vi "Meas Single Record.vi"(7 "sequence item":T1, 8 "error in":errorcluster, 10 "binary data file path (no ext.)":path, 11 "adc session in":T10={"niScope"={"channel cfg"=[], "sessions"=[], "multi cards"=FALSE, "channels"=0, "type"=enum."n/a", "memory [B/chn]"=0, "ext. clock [Hz]"=0.0, "samples count"=0, "use streaming"=FALSE, "proc setup"={"packet size [smpl]"=0, "current timeout [s]"=0.0, "blk2blk timeout [s]"=0.0, "event time"=timestamp(0 s since 1904-01-01), "temp sampl T [s]"=0.0, "data queue"=refnum, "stop notifier"=refnum, "proc ref"=refnum}, "sample width [B]"=0, "ranges [V]"=[], "trigger setup"={"coupling"=1, "level [V]"=0.0, "slope"=0, "mode"=enum."Immediate"}, "fs [Hz]"=0.0, "bitres [bit]"=0, "clock source"=enum."VAL_NO_SOURCE"}, "3458A"={"channels"=[], "sync unit"={"VISA"="", "type"=enum."Picotest U6200A"}, "awg unit"={"type"=enum."Agilent 331xxA to 332xxA", "VISA"="", "enable 10MHz ref"=FALSE}, "sync mode"=enum."MASTER-SLAVE, MASTER clocked by TIMER", "streaming mode"=FALSE, "idn mode"=enum."Auto", "sampling mode"=enum."DCV", "Ts [s]"=0.0, "sample memory [B]"=0, "proc setup"={"channel id"=0, "packet size [smpl]"=0, "current timeout [s]"=0.0, "blk2blk timeout [s]"=0.0, "event time"=timestamp(0 s since 1904-01-01), "stop notifier"=refnum, "data queues"=[], "proc refs"=[], "bus semaphore"=refnum}, "sample size [B]"=0, "sample count"=0, "aux data"={"channel id"=0, "valid?"=[], "gain [V]"=[], "timestamp [s]"=[], "Ts [s]"=0.0, "abs timestamp"=timestamp(0 s since 1904-01-01), "t [deg C]"=[], "multiplex timestamp [s]"=-1.0, "only multiplex?"=FALSE, "multiplex smpl offset"=0}, "ranges [V]"=[], "aperture [s]"=0.0, "LEVEL trigger"={"edge"=enum."POS", "level [V]"=0.0, "coupling"=enum."DC"}, "trigger mode"=enum."AUTO", "measure temp.?"=FALSE, "disp mesages"=[], "shared bus?"=FALSE, "disable display?"=FALSE, "aper mode"=enum."Manual", "aper rules"=[], "multiplex"={"cycles"=0, "delay [s]"=0.0, "enabled"=FALSE, "overhead [s]"=1.0, "tot smpls"=0}}, "dsdll"={"dsdll"={"dsdll path"=path "", "dsdll handle"=[], "output devices"=[], "capture devices"=[]}, "channels"=0, "device id"=0, "channel idns"=[], "proc setup"={"packet size [smpl]"=0, "current timeout [s]"=0.0, "blk2blk timeout [s]"=0.0, "event time"=timestamp(0 s since 1904-01-01), "data queue"=refnum, "stop notifier"=refnum, "proc ref"=refnum}, "samples count"=0, "fs [Hz]"=0.0}, "type"=enum."niScope", "channel idn str"=[], "aux instr idn str"=[], "modified?"=FALSE, "simadc"={"channels"=[], "range [V]"=0.0, "Ts step [s]"=0.0, "time [s]"=0.0, "fs [Hz]"=0.0, "count"=0, "smpl offset"=0, "set count"=0, "bit res"=0}, "force rst?"=FALSE, "exit mode"=enum."Immediate reset", "exit dly"=0.0, "exit tmr"=timestamp(0 s since 1904-01-01), "busy?"=FALSE, "accessed?"=FALSE, "multiplex"={"Type"=enum."Dummy", "gen com ssn"={"visa"="", "primary"=enum."None", "secondary"=enum."None", "channels"=[]}, "delay before [s]"=0.0, "delay post [s]"=0.0, "sequence"=[], "enabled"=FALSE, "ref timestamp [s]"=0.0, "idn string"="", "dev niScope"="", "niScope idx"=0}} {"3458A"."channels"."Range [Vpk]" min=0.0; "niScope"."trigger setup"."level [V]" format="%.2f"; "niScope"."trigger setup"."coupling" items=["AC"=0, "DC"=1, "HF Reject"=3, "LF Reject"=4, "AC Plus HF Reject"=1001]; "niScope"."channel cfg"."Range [Vpk]" min=0.0; "niScope"."channel cfg"."Channel" min=0}) -> (0 "error out":errorcluster, 1 "aborted?":bool, 2 "aux data":T9, 3 "adc session out":T10={"niScope"={"channel cfg"=[], "sessions"=[], "multi cards"=FALSE, "channels"=0, "type"=enum."n/a", "memory [B/chn]"=0, "ext. clock [Hz]"=0.0, "samples count"=0, "use streaming"=FALSE, "proc setup"={"packet size [smpl]"=0, "current timeout [s]"=0.0, "blk2blk timeout [s]"=0.0, "event time"=timestamp(0 s since 1904-01-01), "temp sampl T [s]"=0.0, "data queue"=refnum, "stop notifier"=refnum, "proc ref"=refnum}, "sample width [B]"=0, "ranges [V]"=[], "trigger setup"={"coupling"=1, "level [V]"=0.0, "slope"=0, "mode"=enum."Immediate"}, "fs [Hz]"=0.0, "bitres [bit]"=0, "clock source"=enum."VAL_NO_SOURCE"}, "3458A"={"channels"=[], "sync unit"={"VISA"="", "type"=enum."Picotest U6200A"}, "awg unit"={"type"=enum."Agilent 331xxA to 332xxA", "VISA"="", "enable 10MHz ref"=FALSE}, "sync mode"=enum."MASTER-SLAVE, MASTER clocked by TIMER", "streaming mode"=FALSE, "idn mode"=enum."Auto", "sampling mode"=enum."DCV", "Ts [s]"=0.0, "sample memory [B]"=0, "proc setup"={"channel id"=0, "packet size [smpl]"=0, "current timeout [s]"=0.0, "blk2blk timeout [s]"=0.0, "event time"=timestamp(0 s since 1904-01-01), "stop notifier"=refnum, "data queues"=[], "proc refs"=[], "bus semaphore"=refnum}, "sample size [B]"=0, "sample count"=0, "aux data"={"channel id"=0, "valid?"=[], "gain [V]"=[], "timestamp [s]"=[], "Ts [s]"=0.0, "abs timestamp"=timestamp(0 s since 1904-01-01), "t [deg C]"=[], "multiplex timestamp [s]"=-1.0, "only multiplex?"=FALSE, "multiplex smpl offset"=0}, "ranges [V]"=[], "aperture [s]"=0.0, "LEVEL trigger"={"edge"=enum."POS", "level [V]"=0.0, "coupling"=enum."DC"}, "trigger mode"=enum."AUTO", "measure temp.?"=FALSE, "disp mesages"=[], "shared bus?"=FALSE, "disable display?"=FALSE, "aper mode"=enum."Manual", "aper rules"=[], "multiplex"={"cycles"=0, "delay [s]"=0.0, "enabled"=FALSE, "overhead [s]"=1.0, "tot smpls"=0}}, "dsdll"={"dsdll"={"dsdll path"=path "", "dsdll handle"=[], "output devices"=[], "capture devices"=[]}, "channels"=0, "device id"=0, "channel idns"=[], "proc setup"={"packet size [smpl]"=0, "current timeout [s]"=0.0, "blk2blk timeout [s]"=0.0, "event time"=timestamp(0 s since 1904-01-01), "data queue"=refnum, "stop notifier"=refnum, "proc ref"=refnum}, "samples count"=0, "fs [Hz]"=0.0}, "type"=enum."niScope", "channel idn str"=[], "aux instr idn str"=[], "modified?"=FALSE, "simadc"={"channels"=[], "range [V]"=0.0, "Ts step [s]"=0.0, "time [s]"=0.0, "fs [Hz]"=0.0, "count"=0, "smpl offset"=0, "set count"=0, "bit res"=0}, "force rst?"=FALSE, "exit mode"=enum."Immediate reset", "exit dly"=0.0, "exit tmr"=timestamp(0 s since 1904-01-01), "busy?"=FALSE, "accessed?"=FALSE, "multiplex"={"Type"=enum."Dummy", "gen com ssn"={"visa"="", "primary"=enum."None", "secondary"=enum."None", "channels"=[]}, "delay before [s]"=0.0, "delay post [s]"=0.0, "sequence"=[], "enabled"=FALSE, "ref timestamp [s]"=0.0, "idn string"="", "dev niScope"="", "niScope idx"=0}} {"3458A"."channels"."Range [Vpk]" min=0.0; "niScope"."trigger setup"."level [V]" format="%.2f"; "niScope"."trigger setup"."coupling" items=["AC"=0, "DC"=1, "HF Reject"=3, "LF Reject"=4, "AC Plus HF Reject"=1001]; "niScope"."channel cfg"."Range [Vpk]" min=0.0; "niScope"."channel cfg"."Channel" min=0}, 4 "acquired samples per channel":i64, 6 "record segments info":T8[](array[typedef]))   [LabVIEW 2013]
doc: "This VI initiates sampling of one record with current setup of ADC. It streams the sample data to MAT file of a given path (without extension). The VI also appends logged temperatures to the MAT file. It will return ADC auxiliary data which are valid only if flag 'valid?' in the cluster is True (that should happen all the time except when the sampling was aborted for whatever reason). The VI responds to global stop button called 'btn stop' - it will abort sampling when it is in True state.\n\nIn time multiplexing mode the samples from particular cycles are stored as one stream to the MAT file. Along with them the VI returns 'multiplexing sample offsets', which are zero-based offsets of first sample for each multiplexing cycle."
uses:
  adc/ADC Session.ctl
  drivers/niScope/niScope Session.ctl
  drivers/niScope/niScope Virtual Channel Config.ctl
  drivers/niScope/niScope Virtual Channel Mode.ctl
  drivers/niScope/niScope Virtual Channel Input Z.ctl
  drivers/niScope/niScope Virtual Channel Coupling.ctl
  drivers/niScope/niScope Type.ctl
  drivers/niScope/niScope Digitizing Process Options.ctl
  drivers/niScope/niScope Data Packet.ctl
  drivers/niScope/niScope Trigger Setup.ctl
  <instrlib>/niScope/Controls/niScope trigger coupling.ctl
  <instrlib>/niScope/Controls/niScope trigger slope.ctl
  drivers/niScope/niScope Reference Clock.ctl
  drivers/DMM/3458A Digitizer Session.ctl
  drivers/DMM/3458A Virtual Channel Config.ctl
  drivers/Counter/Counter Session.ctl
  drivers/Counter/Counter Type.ctl
  drivers/AWG/AWG Session.ctl
  drivers/AWG/AWG Type.ctl
  drivers/DMM/3458A Sync Mode.ctl
  drivers/DMM/3458A Idn Mode.ctl
  drivers/DMM/3458A Digitizing Low Levels/Configure/Sampling Mode.ctl
  drivers/DMM/3458A Digitizing Process Options.ctl
  drivers/DMM/3458A Data Packet.ctl
  drivers/DMM/3458A Aux Record Data.ctl
  drivers/DMM/3458A Digitizing Low Levels/Configure/Level Setup.ctl
  drivers/DMM/3458A Digitizing Low Levels/Configure/First Sample Trigger.ctl
  drivers/DMM/3458A Aperture Selection Mode.ctl
  drivers/DMM/3458A Multiplexing Config.ctl
  drivers/dsdll/DSDLL Session.ctl
  drivers/dsdll/dsdll.lvlibp/dsdll_instance.ctl
  drivers/dsdll/dsdll.lvlibp/dsdll_device_record.ctl
  drivers/dsdll/DSDLL Process Config.ctl
  drivers/dsdll/DSDLL Data Packet.ctl
  adc/ADC Type.ctl
  drivers/simulated_adc/SimAdc Config.ctl
  drivers/simulated_adc/SimAdc Channel Cfg.ctl
  adc/ADC On Close Action.ctl
  adc/Multiplexer/MPX Session.ctl
  adc/Multiplexer/MPX Type.ctl
  drivers/Multiplexers/Generic COM/GCOMM Session.ctl
  drivers/Multiplexers/Generic COM/GCOMM Signal.ctl
  drivers/Multiplexers/Generic COM/GCOMM Virtual Channel.ctl
  drivers/Multiplexers/Generic COM/GCOMM Logic State.ctl
  adc/ADC Aux Data.ctl
  adc/Multiplexer/MPX Record Segment Info.ctl
  Meas Sequence Item.ctl
  Meas Sampling Configuration.ctl
  adc/ADC Trig Config.ctl
  adc/ADC Trig Mode Source.ctl
  adc/ADC Trig Coupling.ctl
  adc/ADC Trig Slope.ctl
  processing/QWTB/Meas Proc QWTB Algorithm Parameter Data.ctl
  octave/mat/MAT Type Representation.ctl
  varilib/SGUI Assign Multiple Strings With Tags By Label.vi
  varilib/varilib.lvlib
  drivers/niScope/niScope Virtual Digitizer.lvlib
  drivers/DMM/3458A Virtual Digitizer.lvlib
  drivers/Counter/Counter.lvlib
  drivers/AWG/AWG.lvlib
  drivers/DMM/3458A Digitizing Low Levels/3458A Digitizing Low Levels.lvlib
  drivers/dsdll/dsdll.lvlibp
  drivers/dsdll/DSDLL Virtual Digitizer.lvlib
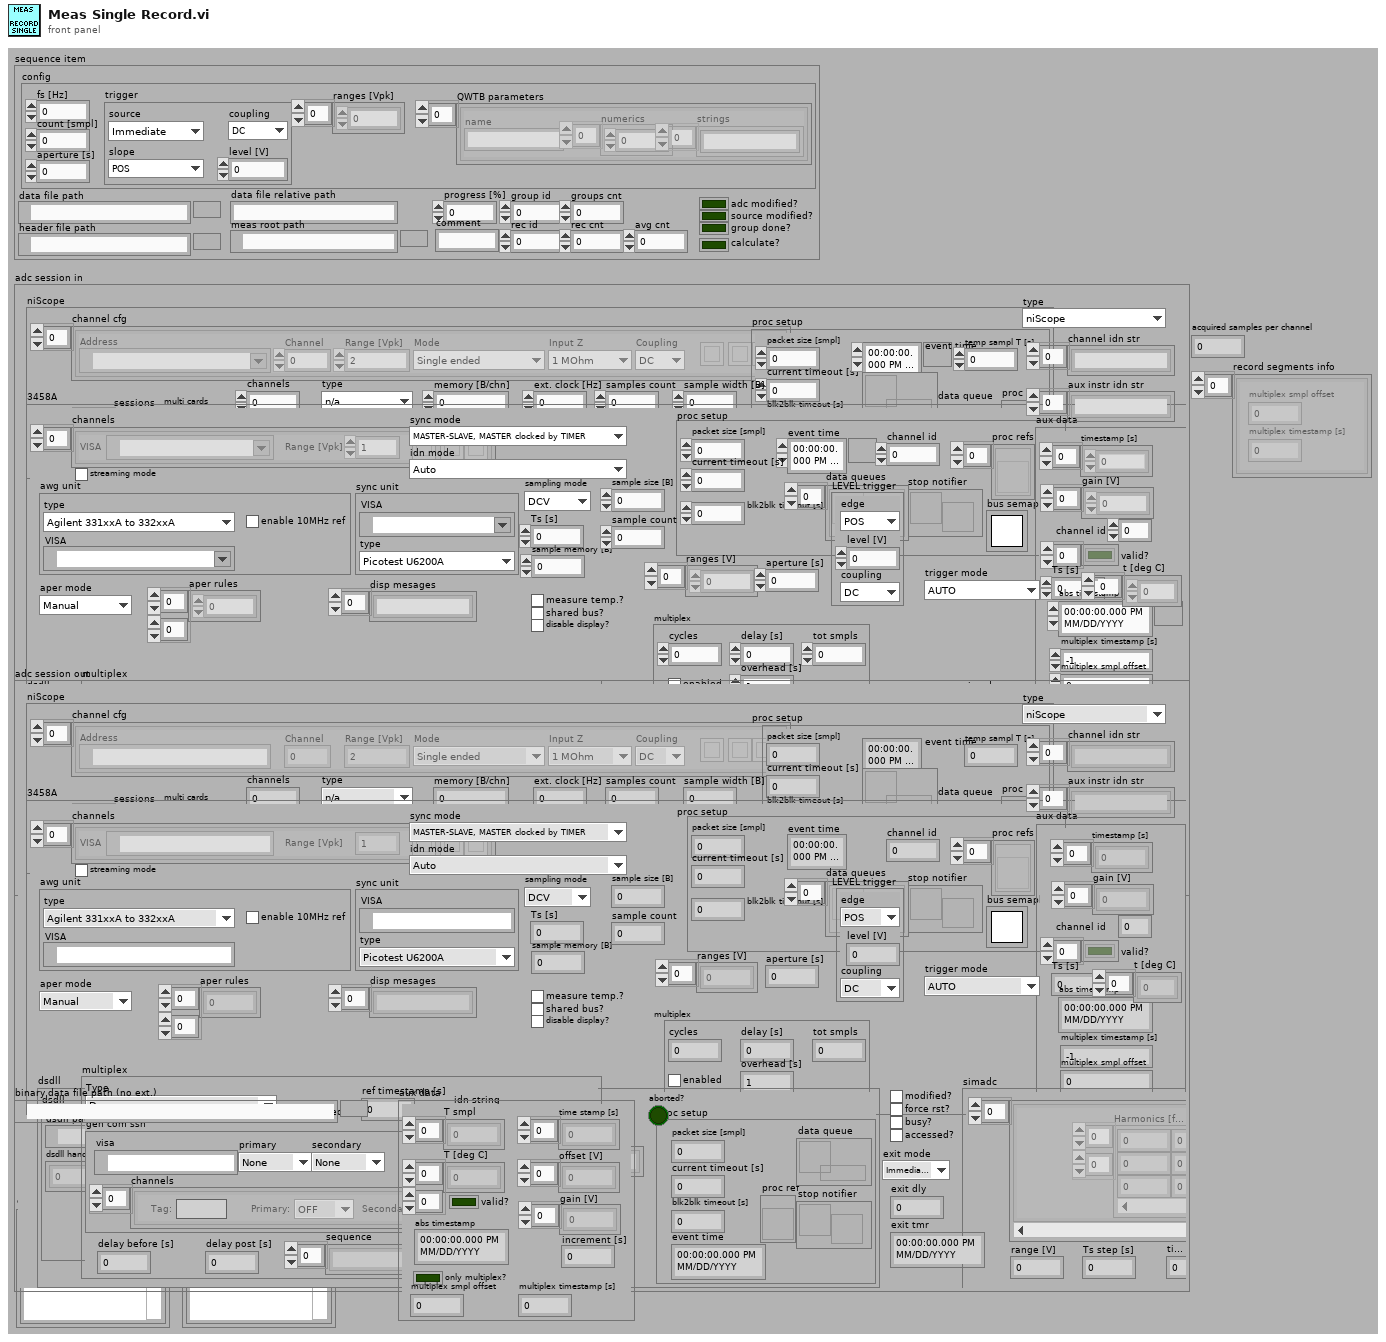
[diagram p1: front panel]
types:
  T1 = typedef "Meas Sequence Item.ctl" = cluster{"config":T2, "data file path":path, "header file path":path, "group id":i32, "rec id":i32, "group done?":bool, "adc modified?":bool, "source modified?":bool, "progress [%]":dbl, "groups cnt":i32, "rec cnt":i32, "data file relative path":string, "meas root path":path, "calculate?":bool, "comment":string, "avg cnt":i32}
  T2 = typedef "Meas Sampling Configuration.ctl" = cluster{"fs [Hz]":dbl, "count [smpl]":i64, "aperture [s]":dbl, "trigger":T3, "ranges [Vpk]":dbl[], "QWTB parameters":T7[]}
  T3 = typedef "ADC Trig Config.ctl" = cluster{"source":T4, "level [V]":dbl, "coupling":T5, "slope":T6}
  T4 = typedef "ADC Trig Mode Source.ctl" = enum16{"Immediate", "External", "Level"}
  T5 = typedef "ADC Trig Coupling.ctl" = enum16{"DC", "AC"}
  T6 = typedef "ADC Trig Slope.ctl" = enum16{"POS", "NEG"}
  T7 = typedef "Meas Proc QWTB Algorithm Parameter Data.ctl" = cluster{"name":string, "numerics":dbl[], "strings":string[]}
  T8 = typedef "MPX Record Segment Info.ctl" = cluster{"multiplex smpl offset":i64, "multiplex timestamp [s]":dbl}
  T9 = typedef "ADC Aux Data.ctl" = cluster{"offset [V]":dbl[], "gain [V]":dbl[], "time stamp [s]":dbl[], "increment [s]":dbl, "T smpl":i64[], "T [deg C]":dbl[][], "valid?":bool, "abs timestamp":timestamp, "only multiplex?":bool, "multiplex smpl offset":i64, "multiplex timestamp [s]":dbl}
  T10 = typedef "ADC Session.ctl" = cluster{"niScope":T11, "3458A":T22, "dsdll":T38, "type":T42, "channel idn str":string[], "aux instr idn str":string[], "modified?":bool, "simadc":T43, "force rst?":bool, "exit mode":T45, "exit dly":dbl, "exit tmr":timestamp, "busy?":bool, "accessed?":bool, "multiplex":T46}
  T11 = typedef "niScope Virtual Digitizer.lvlib/niScope Session.ctl" = cluster{"channel cfg":T12[], "sessions":refnum<k20>[], "multi cards":bool, "channels":i32, "type":T16, "memory [B/chn]":i32, "ext. clock [Hz]":dbl, "samples count":i64, "use streaming":bool, "proc setup":T17, "sample width [B]":i32, "ranges [V]":dbl[], "trigger setup":T18, "fs [Hz]":dbl, "bitres [bit]":i32, "clock source":T21}
  T12 = typedef "niScope Virtual Digitizer.lvlib/niScope Virtual Channel Config.ctl" = cluster{"Address":refnum<k15>, "Channel":i32, "Mode":T13, "Input Z":T14, "Coupling":T15, "Range [Vpk]":dbl, "btn clr":bool, "btn up":bool, "btn down":bool}
  T13 = typedef "niScope Virtual Digitizer.lvlib/niScope Virtual Channel Mode.ctl" = enum16{"Single ended", "Unbal. differential", "Differential"}
  T14 = typedef "niScope Virtual Digitizer.lvlib/niScope Virtual Channel Input Z.ctl" = enum16{"1 MOhm", "50 Ohm"}
  T15 = typedef "niScope Virtual Digitizer.lvlib/niScope Virtual Channel Coupling.ctl" = enum16{"AC", "DC", "GND"}
  T16 = typedef "niScope Virtual Digitizer.lvlib/niScope Type.ctl" = enum16{"n/a", "5922"}
  T17 = typedef "niScope Virtual Digitizer.lvlib/niScope Digitizing Process Options.ctl" = cluster{"packet size [smpl]":i64, "current timeout [s]":dbl, "blk2blk timeout [s]":dbl, "event time":timestamp, "temp sampl T [s]":dbl, "data queue":refnum<queue>, "stop notifier":refnum<notifier>, "proc ref":refnum<vi>}
  T18 = typedef "niScope Virtual Digitizer.lvlib/niScope Trigger Setup.ctl" = cluster{"coupling":T19, "level [V]":dbl, "slope":T20, "mode":enum16{"Immediate", "External", "Level"}}
  T19 = typedef "niScope trigger coupling.ctl" = u16
  T20 = typedef "niScope trigger slope.ctl" = i32
  T21 = typedef "niScope Virtual Digitizer.lvlib/niScope Reference Clock.ctl" = enum16{"VAL_NO_SOURCE", "VAL_CLK_IN", "VAL_PXI_CLOCK", "VAL_EXTERNAL"}
  T22 = typedef "3458A Virtual Digitizer.lvlib/3458A Digitizer Session.ctl" = cluster{"channels":T23[], "sync unit":T24, "awg unit":T26, "sync mode":T28, "streaming mode":bool, "idn mode":T29, "sampling mode":T30, "Ts [s]":dbl, "sample memory [B]":i32, "proc setup":T31, "sample size [B]":i32, "sample count":i32, "aux data":T33, "ranges [V]":dbl[], "aperture [s]":dbl, "LEVEL trigger":T34, "trigger mode":T35, "measure temp.?":bool, "disp mesages":string[], "shared bus?":bool, "disable display?":bool, "aper mode":T36, "aper rules":dbl[][], "multiplex":T37}
  T23 = typedef "3458A Virtual Digitizer.lvlib/3458A Virtual Channel Config.ctl" = cluster{"VISA":refnum<visa-resource-name>, "Range [Vpk]":dbl, "btn clr":bool, "btn up":bool, "btn down":bool}
  T24 = typedef "Counter.lvlib/Counter Session.ctl" = cluster{"VISA":refnum<visa-resource-name>, "type":T25}
  T25 = typedef "Counter.lvlib/Counter Type.ctl" = enum16{"Picotest U6200A", "dummy"}
  T26 = typedef "AWG.lvlib/AWG Session.ctl" = cluster{"type":T27, "VISA":refnum<visa-resource-name>, "enable 10MHz ref":bool}
  T27 = typedef "AWG.lvlib/AWG Type.ctl" = enum16{"Agilent 331xxA to 332xxA", "Agilent 335xxA to 336xxA", "Tektronix AFG3101C", "dummy"}
  T28 = typedef "3458A Virtual Digitizer.lvlib/3458A Sync Mode.ctl" = enum16{"MASTER-SLAVE, MASTER clocked by TIMER", "MASTER-SLAVE, MASTER clocked by AWG", "ALL clocked by AWG", "MASTER-SLAVE, ALL clocked by TIMER", "ALL clocked by AWG with DFLL"}
  T29 = typedef "3458A Virtual Digitizer.lvlib/3458A Idn Mode.ctl" = enum16{"Auto", "Sequential (chn A, chn B, ...)", "From calibration string"}
  T30 = typedef "3458A Virtual Digitizer.lvlib/3458A Digitizing Low Levels.lvlib/Sampling Mode.ctl" = enum16{"DCV", "DSDC", "DSAC"}
  T31 = typedef "3458A Virtual Digitizer.lvlib/3458A Digitizing Process Options.ctl" = cluster{"channel id":i32, "packet size [smpl]":i32, "current timeout [s]":dbl, "blk2blk timeout [s]":dbl, "event time":timestamp, "stop notifier":refnum<notifier>, "data queues":refnum<queue>[], "proc refs":refnum<vi>[], "bus semaphore":T32}
  T32 = typedef "Semaphore RefNum" = refnum<k1>
  T33 = typedef "3458A Virtual Digitizer.lvlib/3458A Aux Record Data.ctl" = cluster{"channel id":i32, "valid?":bool[], "gain [V]":dbl[], "timestamp [s]":dbl[], "Ts [s]":dbl, "abs timestamp":timestamp, "t [deg C]":dbl[], "multiplex timestamp [s]":dbl, "only multiplex?":bool, "multiplex smpl offset":i64}
  T34 = typedef "3458A Virtual Digitizer.lvlib/3458A Digitizing Low Levels.lvlib/Level Setup.ctl" = cluster{"edge":enum16{"POS", "NEG"}, "level [V]":dbl, "coupling":enum16{"DC", "AC"}}
  T35 = typedef "3458A Virtual Digitizer.lvlib/3458A Digitizing Low Levels.lvlib/First Sample Trigger.ctl" = enum16{"AUTO", "EXT", "SYN", "SGL", "HOLD", "LEVEL"}
  T36 = typedef "3458A Virtual Digitizer.lvlib/3458A Aperture Selection Mode.ctl" = enum16{"Manual", "Maximum", "Table"}
  T37 = typedef "3458A Multiplexing Config.ctl" = cluster{"cycles":i32, "delay [s]":dbl, "enabled":bool, "overhead [s]":dbl, "tot smpls":i64}
  T38 = typedef "DSDLL Virtual Digitizer.lvlib/DSDLL Session.ctl" = cluster{"dsdll":T39, "channels":i32, "device id":i32, "channel idns":string[], "proc setup":T41, "samples count":i32, "fs [Hz]":dbl}
  T39 = typedef "dsdll.lvlibp/dsdll_instance.ctl" = cluster{"dsdll path":path, "dsdll handle":u8[], "output devices":T40[], "capture devices":T40[]}
  T40 = typedef "dsdll.lvlibp/dsdll_device_record.ctl" = cluster{"guid":u8[], "name":string}
  T41 = typedef "DSDLL Virtual Digitizer.lvlib/DSDLL Process Config.ctl" = cluster{"packet size [smpl]":i32, "current timeout [s]":dbl, "blk2blk timeout [s]":dbl, "event time":timestamp, "data queue":refnum<queue>, "stop notifier":refnum<notifier>, "proc ref":refnum<vi>}
  T42 = typedef "ADC Type.ctl" = enum16{"niScope", "3458A", "DirectSound DLL", "dummy"}
  T43 = typedef "SimAdc Config.ctl" = cluster{"channels":T44[], "range [V]":dbl, "Ts step [s]":dbl, "time [s]":dbl, "fs [Hz]":dbl, "count":i64, "smpl offset":i64, "set count":i64, "bit res":i32}
  T44 = typedef "SimAdc Channel Cfg.ctl" = cluster{"harmonics":dbl[][], "btn clear":bool, "noise":dbl, "fundamental [Hz]":dbl}
  T45 = typedef "ADC On Close Action.ctl" = enum16{"Immediate reset", "Delayed reset"}
  T46 = typedef "MPX Session.ctl" = cluster{"Type":T47, "gen com ssn":T48, "delay before [s]":dbl, "delay post [s]":dbl, "sequence":string[], "enabled":bool, "ref timestamp [s]":dbl, "idn string":string, "dev niScope":refnum<k15>, "niScope idx":i32}
  T47 = typedef "MPX Type.ctl" = enum16{"Dummy", "Generic - COM port", "Generic - niScope PFI"}
  T48 = typedef "GCOMM Session.ctl" = cluster{"visa":refnum<visa-resource-name>, "primary":T49, "secondary":T49, "channels":T50[]}
  T49 = typedef "GCOMM Signal.ctl" = enum16{"None", "DTR", "RTS"}
  T50 = typedef "GCOMM Virtual Channel.ctl" = cluster{"Primary:":T51, "Secondary:":T51, "btn clr":bool, "btn up":bool, "btn down":bool, "Tag:":string}
  T51 = typedef "GCOMM Logic State.ctl" = enum16{"OFF", "ON"}
  T52 = typedef "MAT Type Representation.ctl" = enum16{"DBL", "SGL", "I32", "I16", "U16", "U8", "CDB", "CSG", "STR"}
  T53 = typedef "ADC Current Configuration.ctl" = cluster{"count [smpl]":i64, "channels count":i32, "fs [Hz]":dbl, "ranges [V]":dbl[], "trigger":T3, "ext freq. locked?":bool, "streaming on?":bool, "is int16?":bool, "bitres":i32}
  T54 = typedef "Meas Samples Stream.ctl" = cluster{"file ref":refnum<file>, "data offset [B]":i64, "var offset [B]":i64, "data type":T52, "written smpls":i64, "channels":i64}
  T55 = typedef "ADC Data Packet.ctl" = cluster{"int32":i32[][], "int16":i16[][], "offset [smpl]":i64, "count [smpl]":i32, "is int16?":bool, "all done?":bool, "sampling?":bool, "instr buffer [%]":dbl, "queue buffer [%]":dbl, "valid?":bool}
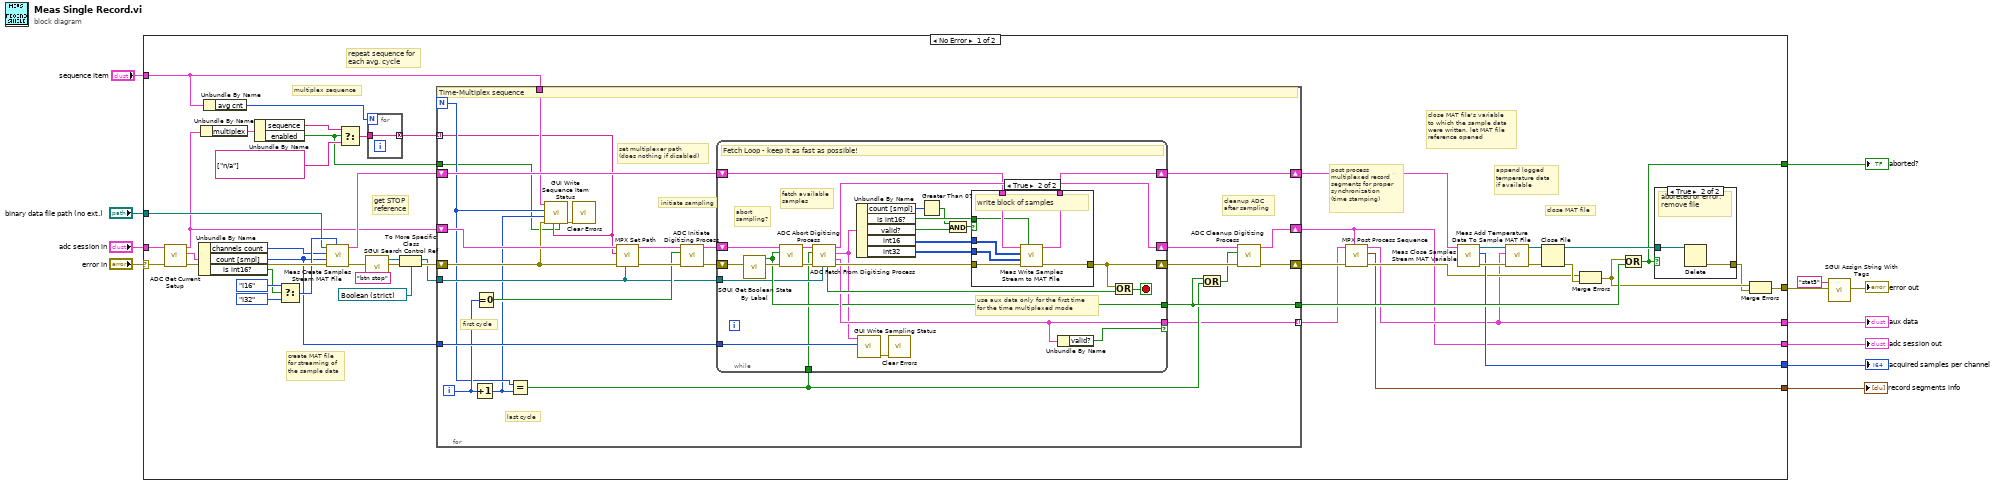
[diagram p0: block diagram]
diagram:
  n1 = case shown="No Error" "error in" {
    selector: "error in" -> [w46 w126]
    tunnel: "adc session in" -> [w59 w125]
    tunnel: "binary data file path (no ext.)" -> [w54 _]
    tunnel: [w41 w126] -> w5
    tunnel: [w18 w125] -> w9
    tunnel: [w20 _] -> w8
    tunnel: [w40 _] -> w7
    tunnel: [w37 _] -> w6
    tunnel: [w19 _] -> w2
    tunnel: "sequence item" -> [w14 _]
    frame No Error {
      # "repeat sequence for\neach avg. cycle"
      # "post process\nmultiplexed record\nsegments for proper\nsynchronization\n(time stamping)"
      # "get STOP\nreference"
      # "multiplex sequence"
      # "close MAT file"
      # "append logged\ntemperature data\nif available"
      # "close MAT file's variable\nto which the sample data\nwere written, let MAT file\nreference opened"
      # "create MAT file\nfor streaming of\nthe sample data"
      n2 = call "ADC Get Current Setup.vi"("error in"=w46, "adc session in"=w59) -> ("error out"=w58:errorcluster, "common attributes"=w39:T53, "adc session out"=w34:T10)  [unwired: 6 in, 1 out]
      n3 = Unbundle By Name(w39) -> ("channels count"=w36:i32, "count [smpl]"=w35:i64, "is int16?"=w38:bool)
      n4 = Unbundle By Name(w34) -> ("multiplex"=w33:T46)
      n5 = Unbundle By Name(w14) -> ("avg cnt"=w17:i32)
      n6 = Unbundle By Name(w33) -> ("sequence"=w32:string[], "enabled"=w13:bool)
      n7 = Select(t=MAT_Type_Representation."I16" ("data type"), s=w38, f=MAT_Type_Representation."I32" ("data type")) -> (s? t:f=w55:T52)
      n8 = call "Meas Create Samples Stream MAT File.vi"("data type"=w55, "error in"=w58, "samples count"=w35, "channels count"=w36, "binary data file path"=w54) -> ("error out"=w29:errorcluster, "stream session"=w53:T54)  [unwired: 5 in]
      n9 = Select(t=w32, s=w13, f=string[] ["n/a"]) -> (s? t:f=w16:string[])
      n10 = call "SGUI Search Control Ref.vi"("error in"=w29, "control label (empty)"="btn stop") -> ("error out"=w28:errorcluster, "control ref out"=w26:refnum<vi>)  [unwired: 7 in, 1 out]
      n11 = for {
        N: w17 -> [_]
        tunnel: [w60] -> w15 mode=concatenating
        tunnel: w16 -> [w60]
      }
      n12 = To More Specific Class(target class=refnum<vi> refnum ("OK Button"), reference=w26, error in=w28) -> (specific class reference=w25:refnum<vi>, error out=w27:errorcluster)
      n13 = for {
        N -> [w64]
        tunnel: [w70] -> w21 mode=indexing
        tunnel: [w74] -> w45
        tunnel: w35 -> [w82]
        shift-right: [w83] -> w23
        shift-left: w27 -> [w66]
        shift-right: [w84] -> w18
        shift-left: w34 -> [w69]
        shift-right: [w85] -> w52
        shift-left: w53 -> [w86]
        tunnel: w15 -> [w62] mode=indexing
        tunnel: w25 -> [w75]
        tunnel: w14 -> [w65]
        tunnel: w13 -> [w61]
        i -> [w76]
        # "last cycle"
        # "first cycle"
        # "set multiplexer path\n(does nothing if disabled)"
        # "cleanup ADC \nafter sampling"
        # "initiate sampling"
        # "Time-Multiplex sequence"
        n14 = Increment(x=w76) -> (x+1=w63:i32)
        n15 = Equal To 0?(x=w76) -> (x = 0?=w77:bool)
        n16 = Equal?(x=w64, y=w63) -> (x = y?=w71:bool)
        n17 = call "GUI Write Sequence Item Status.vi"("multiplex enabled (False)"=w61, "multiplex tag"=w62, "error in"=w66, "sub-rec id"=w63, "sub-rec count"=w64, "sequence item"=w65) -> ("error out"=w67:errorcluster)  [unwired: 4 in, 1 out]
        n18 = call <vilib>:"Clear Errors.vi"("error in (no error)"=w67) -> ()  [unwired: 6 in, 1 out]
        n19 = call "MPX Set Path.vi"("stop ref"=w75, "error in"=w66, "path"=w62, "session in"=w69) -> ("error out"=w78:errorcluster, "session out"=w68:T10)  [unwired: 6 in]
        n20 = call "ADC Initiate Digitizing Process.vi"("error in"=w78, "Is first multiplex cycle? (True)"=w77, "adc session in"=w68) -> ("error out"=w72:errorcluster, "adc session out"=w81:T10)  [unwired: 7 in]
        n21 = while {
          shift-right: [w99] -> w80
          shift-left: w72 -> [w113]
          shift-right: [w108] -> w79
          shift-left: w81 -> [w111]
          shift-right: [w103] -> w85
          shift-left: w86 -> [w104]
          tunnel: [w98] -> w70 if=w87
          tunnel: [w97] -> w74
          tunnel: w82 -> [w91]
          tunnel: w75 -> [w89]
          tunnel: w71 -> [w88]
          stop <- w106 stop-if-true
          # "use aux data only for the first time\nfor the time multiplexed mode"
          # "fetch available\nsamples"
          # "abort\nsampling?"
          # "Fetch Loop - keep it as fast as possible!"
          n22 = call "SGUI Get Boolean State By Label.vi"("error in"=w113) -> ("error out"=w112:errorcluster, "binary state out"=w97:bool)  [unwired: 8 in, 1 out]
          n23 = call "ADC Abort Digitizing Process.vi"("error in"=w112, "send abort signal? (True)"=w97, "adc session in"=w111) -> ("error out"=w110:errorcluster, "adc session out"=w109:T10)  [unwired: 7 in]
          n24 = call "ADC Fetch From Digitizing Process.vi"("stop ref"=w89, "error in"=w110, "Is last multiplexing cycle? (True)"=w88, "adc session in"=w109) -> ("error out"=w105:errorcluster, "aux data"=w98:T9, "data packet"=w92:T55, "adc session out"=w108:T10, "fetching done?"=w107:bool)  [unwired: 3 in]
          n25 = Unbundle By Name(w92) -> ("count [smpl]"=w96:i32, "is int16?"=w100:bool, "valid?"=w93:bool, "int16"=w102:i16[][], "int32"=w101:i32[][])
          n26 = call "GUI Write Sampling Status.vi"("total samples"=w91, "data"=w92) -> ("error out"=w90:errorcluster)  [unwired: 9 in]
          n27 = call <vilib>:"Clear Errors.vi"("error in (no error)"=w90) -> ()  [unwired: 6 in, 1 out]
          n28 = Greater Than 0?(x=w96) -> (x > 0?=w94:bool)
          n29 = Compound Arithmetic op=AND(w94, w93) -> (w95:bool)
          n30 = case shown="True" w95 {
            tunnel: w105 -> [w115 w122]
            tunnel: w104 -> [w114 w121]
            tunnel: [w114 w120] -> w103
            tunnel: w102 -> [_ w119]
            tunnel: w101 -> [_ w118]
            tunnel: w100 -> [_ w117]
            tunnel: [w115 w116] -> w99
            frame False {
              # "no data available"
            }
            frame True {
              # "write block of samples"
              n31 = call "Meas Write Samples Stream to MAT File.vi"("is int16?"=w117, "error in"=w122, "int32"=w118, "int16"=w119, "stream session in"=w121) -> ("error out"=w116:errorcluster, "stream session out"=w120:T54)  [unwired: 5 in]
            }
          }
          n32 = Unbundle By Name(w98) -> ("valid?"=w87:bool)
          n33 = Compound Arithmetic op=OR(w99, w107) -> (w106:bool)
        }
        n34 = Compound Arithmetic op=OR(w74, w71) -> (w73:bool)
        n35 = call "ADC Cleanup Digitizing Process.vi"("error in"=w80, "Last multiplex cycle? (True)"=w73, "adc session in"=w79) -> ("error out"=w83:errorcluster, "adc session out"=w84:T10)  [unwired: 7 in]
      }
      n36 = call "MPX Post Process Sequence.vi"("adc session in"=w18, "error in"=w23, "aux data of particular records in mpx sequence"=w21) -> ("error out"=w22:errorcluster, "record segment offset"=w19:T8[], "aux data"=w20:T9)  [unwired: 6 in]
      n37 = call "Meas Close Samples Stream MAT Variable.vi"("stream session"=w52) -> ("error out"=w51:errorcluster, "written samples"=w37:i64, "MAT file ref out"=w50:refnum<file>)  [unwired: 8 in]
      n38 = call "Meas Add Temperature Data To Sample MAT File.vi"("error in"=w51, "aux data"=w20, "MAT file ref in"=w50) -> ("error out"=w49:errorcluster, "MAT file ref out"=w48:refnum<file>)  [unwired: 7 in]
      n39 = Close File(refnum=w48, error in=w49) -> (path=w44:path, error out=w47:errorcluster)
      n40 = Merge Errors(w22, w47) -> (w43:errorcluster)
      n41 = Compound Arithmetic op=OR(w43, w45) -> (w40:bool)
      n42 = case shown="True" w40 {
        tunnel: w44 -> [_ w124]
        tunnel: [_ w123] -> w42
        frame False {
        }
        frame True {
          # "aboreted or error:\nremove file"
          n43 = Delete(path (use dialog)=w124) -> (error out=w123:errorcluster)  [unwired: 4 in, 2 out]
        }
      }
      n44 = Merge Errors(w43, w42) -> (w41:errorcluster)
    }
    frame Error {
    }
  }
  "adc session out" <- w9
  "aux data" <- w8
  "aborted?" <- w7
  "acquired samples per channel" <- w6
  "record segments info" <- w2
  n45 = call-poly "SGUI Assign String With Tags.vi"("error in"=w5, "label(s) (empty)"="stat3") -> ("error out"=→"error out":errorcluster)  [unwired: 8 in, 1 out]
